vi "SRV_Get Data Subset for Display.vi"(0 "All Motor Control Config":T1[](array[typedef]) {"Release Cmds"."Motor Control Commands Array"."Value" format="%02x"; "Release Cmds"."Motor Control Commands Array"."Register" format="%02x"; "Release Cmds"."Motor Control Commands Array"."I2C Address" format="%02x"; "Press Cmds"."Motor Control Commands Array"."Value" format="%02x"; "Press Cmds"."Motor Control Commands Array"."Register" format="%02x"; "Press Cmds"."Motor Control Commands Array"."I2C Address" format="%02x"}, 5 "Register refs":refnum<vi>[](array[refnum]), 11 "error in (no error)":errorcluster, 12 "Row Start Index":i32, 13 "Number of Rows to Display (3)":i32=3) -> (4 "All Motor Control Config dup":T1[](array[typedef]) {"Release Cmds"."Motor Control Commands Array"."Value" format="%02x"; "Release Cmds"."Motor Control Commands Array"."Register" format="%02x"; "Release Cmds"."Motor Control Commands Array"."I2C Address" format="%02x"; "Press Cmds"."Motor Control Commands Array"."Value" format="%02x"; "Press Cmds"."Motor Control Commands Array"."Register" format="%02x"; "Press Cmds"."Motor Control Commands Array"."I2C Address" format="%02x"}, 6 "Motor Control Config GUI":T6={"Motor Control Button Index 0"={"Button Name"="Button xx", "Button Label"="", "Motor Type"=enum."Servo", "Press Cmds"={"Motor Control Commands Array"=[]}, "Release Cmds"={"Motor Control Commands Array"=[]}, "Icon"=0}, "Motor Control Button Index 1"={"Button Name"="Button xx", "Button Label"="", "Motor Type"=enum."Servo", "Press Cmds"={"Motor Control Commands Array"=[]}, "Release Cmds"={"Motor Control Commands Array"=[]}, "Icon"=0}, "Motor Control Button Index 2"={"Button Name"="Button xx", "Button Label"="", "Motor Type"=enum."Servo", "Press Cmds"={"Motor Control Commands Array"=[]}, "Release Cmds"={"Motor Control Commands Array"=[]}, "Icon"=0}} {"Motor Control Button Index 2"."Release Cmds"."Motor Control Commands Array"."Value" format="%02x"; "Motor Control Button Index 2"."Release Cmds"."Motor Control Commands Array"."Register" format="%02x"; "Motor Control Button Index 2"."Release Cmds"."Motor Control Commands Array"."I2C Address" format="%02x"; "Motor Control Button Index 2"."Press Cmds"."Motor Control Commands Array"."Value" format="%02x"; "Motor Control Button Index 2"."Press Cmds"."Motor Control Commands Array"."Register" format="%02x"; "Motor Control Button Index 2"."Press Cmds"."Motor Control Commands Array"."I2C Address" format="%02x"; "Motor Control Button Index 1"."Release Cmds"."Motor Control Commands Array"."Value" format="%02x"; "Motor Control Button Index 1"."Release Cmds"."Motor Control Commands Array"."Register" format="%02x"; "Motor Control Button Index 1"."Release Cmds"."Motor Control Commands Array"."I2C Address" format="%02x"; "Motor Control Button Index 1"."Press Cmds"."Motor Control Commands Array"."Value" format="%02x"; "Motor Control Button Index 1"."Press Cmds"."Motor Control Commands Array"."Register" format="%02x"; "Motor Control Button Index 1"."Press Cmds"."Motor Control Commands Array"."I2C Address" format="%02x"; "Motor Control Button Index 0"."Release Cmds"."Motor Control Commands Array"."Value" format="%02x"; "Motor Control Button Index 0"."Release Cmds"."Motor Control Commands Array"."Register" format="%02x"; "Motor Control Button Index 0"."Release Cmds"."Motor Control Commands Array"."I2C Address" format="%02x"; "Motor Control Button Index 0"."Press Cmds"."Motor Control Commands Array"."Value" format="%02x"; "Motor Control Button Index 0"."Press Cmds"."Motor Control Commands Array"."Register" format="%02x"; "Motor Control Button Index 0"."Press Cmds"."Motor Control Commands Array"."I2C Address" format="%02x"}, 15 "error out":errorcluster)   [LabVIEW 2009]
doc: "Author: Mike Schultz (LogicPD, Inc)"
uses:
  SRV_Motor Control Button Config.ctl
  SRV_Motor Legos-Servo.ctl
  SRV_Motor Control Commands Cluster.ctl
  SRV_Motor Control Command Config.ctl
  SRV_Motor Control Button Icons_FALSE.ctl
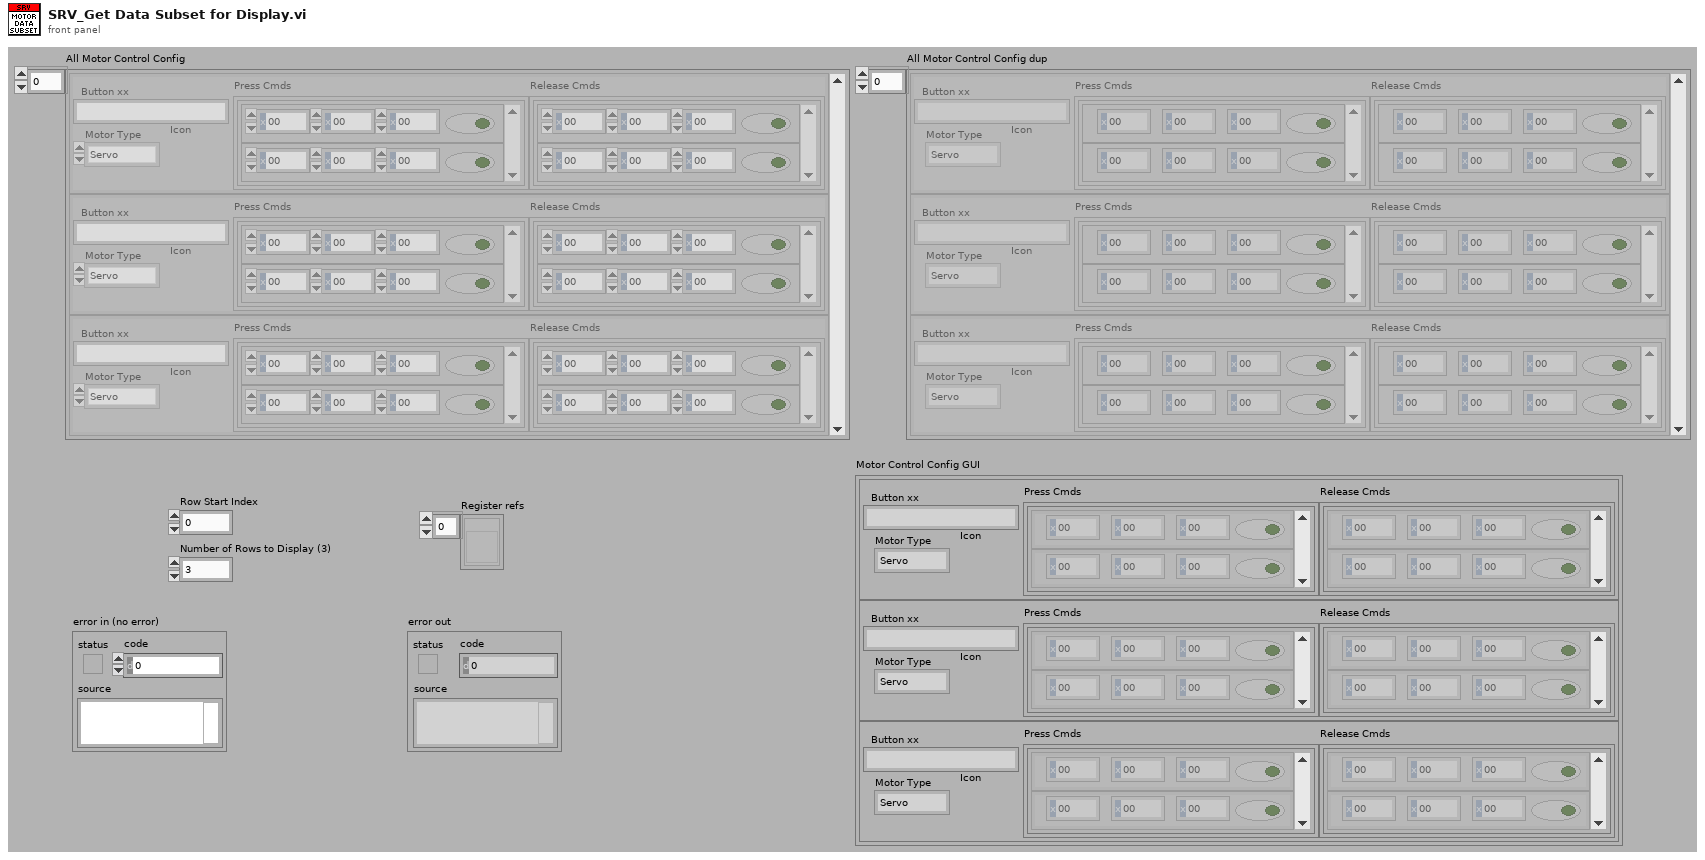
[diagram p1: front panel]
types:
  T1 = typedef "SRV_Motor Control Button Config.ctl" = cluster{"Button Name":string, "Button Label":string, "Motor Type":T2, "Press Cmds":T3, "Release Cmds":T3, "Icon":T5}
  T2 = typedef "SRV_Motor Legos-Servo.ctl" = enum16{"Servo", "Legos", "Shared Var"}
  T3 = typedef "SRV_Motor Control Commands Cluster.ctl" = cluster{"Motor Control Commands Array":T4[]}
  T4 = typedef "SRV_Motor Control Command Config.ctl" = cluster{"I2C Address":u8, "Register":u8, "Value":u8, "Active":bool}
  T5 = typedef "SRV_Motor Control Button Icons_FALSE.ctl" = u16
  T6 = cluster{"Motor Control Button Index 0":T1, "Motor Control Button Index 1":T1, "Motor Control Button Index 2":T1}
  T7 = enum8{"Enabled", "Disabled", "Disabled and Grayed Out"}
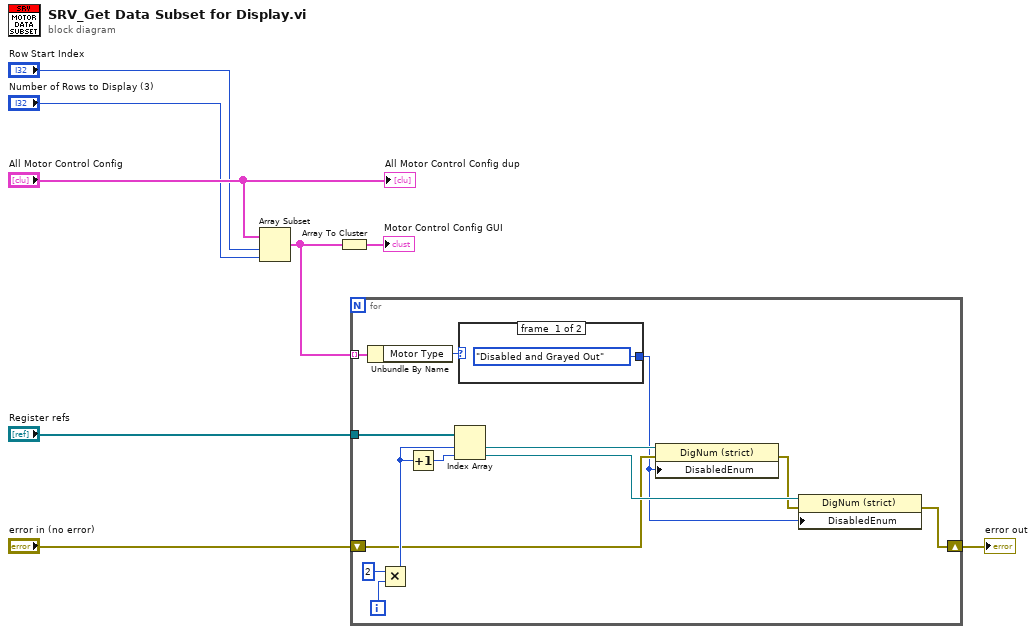
[diagram p0: block diagram]
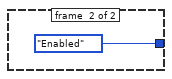
[diagram p2: hidden frame]
diagram:
  n1 = Array Subset(array="All Motor Control Config", index="Row Start Index", length="Number of Rows to Display (3)") -> (w4:T1[])
  n2 = Array To Cluster(array=w4) -> (cluster=→"Motor Control Config GUI":cluster{"[0]":T1, "[1]":T1, "[2]":T1})
  n3 = for {
    tunnel: w4 -> [w21] mode=indexing
    tunnel: "Register refs" -> [w17]
    shift-right: [w11] -> w2
    shift-left: "error in (no error)" -> [w10]
    i -> [w19]
    n4 = Unbundle By Name(w21) -> ("Motor Type"=w20:T2)
    n5 = Multiply(x=2, y=w19) -> (x*y=w16:i32)
    n6 = Increment(x=w16) -> (x+1=w15:i32)
    n7 = Index Array(array=w17, index #1=w16, index #2=w15) -> (element #1=w14:refnum<vi>, element #2=w13:refnum<vi>)
    n8 = case shown="\"Shared Var\"" w20 {
      tunnel: [T7."Disabled and Grayed Out" ("Disabled") T7."Enabled" ("Disabled")] -> w9
      frame #0 {
      }
      frame #1 {
      }
    }
    n9 = property class="DigNum (strict)"(reference=w14, error in=w10, "DisabledEnum"=w9) -> (error out=w12:errorcluster)  [unwired: 1 out]
    n10 = property class="DigNum (strict)"(reference=w13, error in=w12, "DisabledEnum"=w9) -> (error out=w11:errorcluster)  [unwired: 1 out]
  }
  "error out" <- w2
  "All Motor Control Config dup" <- "All Motor Control Config"
